vi "Manual_Cool_Heat.vi"(8 "error in":errorcluster, 11 "input cluster":T3={"Core"={"Current VI Reference"=refnum, "Close Panel on Exit?"=FALSE, "Exit"=FALSE, "Initialized?"=FALSE}, "Connections"={"cDAQ"={"Task"="", "Connected"=TRUE, "Active"=TRUE, "ID"=""}, "Camera"={"Session"="16511205", "Connected"=TRUE, "Active"=FALSE, "Placeholder"=refnum}, "PSU"={"Port"="", "Connected"=FALSE, "Active"=FALSE}, "Arduino"={"Port"="", "Connected"=FALSE, "Active"=FALSE}}, "Data Acquisition"={"Setup"={"Label"="Sample", "Operator"="N/A", "Notes"="", "TempGrad"=-1.0, "TargetTemp"=-30.0, "Sample Volume"=1.0}, "Camera"={"Image"=refnum, "Save Image"=refnum, "Image Frequency"=20, "Rectangle"={"Left"=163, "Top"=40, "Right"=1653, "Bottom"=1024, "Rotation"=0.0}, "Calibration"={"Top Left"={"X"=0.0, "Y"=0.0}, "Top Right"={"X"=0.0, "Y"=0.0}, "Bottom Left"={"X"=0.0, "Y"=0.0}, "Bottom Right"={"X"=0.0, "Y"=0.0}, "Fixpoint"={"X"=0.0, "Y"=0.0}, "Scan Area"=0.0, "Fixpoint Area"=0.0, "Well Pixels"=[], "Valid"=FALSE}, "FocusPos"=0, "Display Mapping"=10}, "Thermistor"={"Sample Size"=3, "Calibration"={"B0.100"=[3746.6, 3750.1, 3743.8, 3749.4, 3745.3, 3741.2, 3742.3, 3742.5], "R25"=[2.2535, 2.2652, 2.2631, 2.2631, 2.2631, 2.2501, 2.2549, 2.2676], "c"=[[-1.735921, 1.0956271, -0.2334593, 0.0229947, -0.0009224], [-2.1276337, 1.4006174, -0.3194056, 0.0337046, -0.0014085], [-2.1731341, 1.4499599, -0.3370628, 0.036201, -0.0015282], [-2.0647232, 1.3741488, -0.3194613, 0.0344214, -0.0014593], [-2.356994, 1.6319471, -0.3929067, 0.0428522, -0.0017977], [-2.0427871, 1.4165762, -0.345474, 0.0385267, -0.0016538], [-2.1725266, 1.4989325, -0.3661616, 0.0412033, -0.0017892], [-2.2048521, 1.4601067, -0.3370514, 0.0360935, -0.0015259]], "State"=[FALSE, TRUE, TRUE, TRUE, FALSE, FALSE, FALSE, FALSE], "V_S"=12.004, "R_S"=10.0}, "Timing Mode"=14713}, "Partition"={"Data"=[], "Cell Label"="", "Cell Color"=0, "Height"=10, "Width"=16, "Grid"=[]}, "Queue"={"Size"=10, "Queue"=refnum}, "Sample Rate"=120, "Active"=FALSE, "Ready"=TRUE, "Graph Mode"=0, "Gradient Buffer"=2}, "Control"={"Sample Rate"=1, "PID gains"={"proportional gain (Kc)"=7.56364319842873, "integral time (Ti, min)"=0.13615714612774, "derivative time (Td, min)"=0.0301129593449614}}, "Manual Temp Control"={"TargetTemp"=1.0, "Mode"=0, "Active"=FALSE}} {"Manual Temp Control"."Mode" items=["Cool", "Heat"]; "Manual Temp Control"."TargetTemp" min=-40.0 max=40.0 step=0.5 format="%#_g °C"; "Control"."PID gains"."derivative time (Td, min)" format="%.3f"; "Control"."PID gains"."integral time (Ti, min)" format="%.3f"; "Control"."PID gains"."proportional gain (Kc)" format="%.3f"; "Control"."Sample Rate" min=1 max=20 step=1 format="%.0f Samples/sec"; "Data Acquisition"."Gradient Buffer" min=2 max=30 step=1; "Data Acquisition"."Graph Mode" items=["Thermistor Temperature", "Camera Temperature"]; "Data Acquisition"."Thermistor"."Timing Mode" items=["Automatic"=16097, "High Resolution"=10195, "High Speed"=14712, "Best 50 Hz Rejection"=14713, "Best 60 Hz Rejection"=14714, "Custom"=10137]; "Data Acquisition"."Thermistor"."Calibration"."R_S" min=0.1 max=1000.0 format="%#_g kOhm"; "Data Acquisition"."Thermistor"."Calibration"."V_S" min=5.0 max=48.0 format="%#_g V"; "Data Acquisition"."Thermistor"."Calibration"."R25" min=0.1 max=1000.0 format="%#_g kOhm"; "Data Acquisition"."Thermistor"."Calibration"."B0.100" min=100.0 max=10000.0 format="%#_g K"; "Data Acquisition"."Thermistor"."Sample Size" min=1 max=200; "Data Acquisition"."Sample Rate" min=20 max=240 format="%.0f samples/min"; "Data Acquisition"."Queue"."Size" min=1 max=200; "Data Acquisition"."Camera"."Display Mapping" items=["Default"=10, "Most Significant Bits"=11, "Full Dynamic"=12, "Downshift"=13, "Given Range"=14, "90% Dynamic"=15, "Given Percent Range"=16]; "Data Acquisition"."Camera"."Calibration"."Fixpoint"."Y" format="%.2f"; "Data Acquisition"."Camera"."Calibration"."Fixpoint"."X" format="%.2f"; "Data Acquisition"."Camera"."Calibration"."Top Left"."Y" format="%.2f"; "Data Acquisition"."Camera"."Calibration"."Top Left"."X" format="%.2f"; "Data Acquisition"."Camera"."Calibration"."Top Right"."Y" format="%.2f"; "Data Acquisition"."Camera"."Calibration"."Top Right"."X" format="%.2f"; "Data Acquisition"."Camera"."Calibration"."Bottom Left"."Y" format="%.2f"; "Data Acquisition"."Camera"."Calibration"."Bottom Left"."X" format="%.2f"; "Data Acquisition"."Camera"."Calibration"."Bottom Right"."Y" format="%.2f"; "Data Acquisition"."Camera"."Calibration"."Bottom Right"."X" format="%.2f"; "Data Acquisition"."Camera"."Rectangle"."Rotation" min=-90.0 max=90.0 step=1.0 format="%.2f"; "Data Acquisition"."Camera"."Rectangle"."Left" scale=0.0..1024.0; "Data Acquisition"."Camera"."Rectangle"."Right" scale=0.0..1024.0; "Data Acquisition"."Camera"."Image Frequency" min=1 max=60 step=1; "Data Acquisition"."Setup"."Sample Volume" min=0.0 max=500.0 format="%#_g µL"; "Data Acquisition"."Setup"."TargetTemp" min=-40.0 max=40.0 step=0.5 format="%#_g °C"; "Data Acquisition"."Setup"."TempGrad" min=-100.0 max=100.0 step=0.1 format="%#_g °C/min"}) -> (0 "error out":errorcluster, 2 "State out":string, 3 "input cluster out":T3={"Core"={"Current VI Reference"=refnum, "Close Panel on Exit?"=FALSE, "Exit"=FALSE, "Initialized?"=FALSE}, "Connections"={"cDAQ"={"Task"="", "Connected"=TRUE, "Active"=TRUE, "ID"=""}, "Camera"={"Session"="16511205", "Connected"=TRUE, "Active"=FALSE, "Placeholder"=refnum}, "PSU"={"Port"="", "Connected"=FALSE, "Active"=FALSE}, "Arduino"={"Port"="", "Connected"=FALSE, "Active"=FALSE}}, "Data Acquisition"={"Setup"={"Label"="Sample", "Operator"="N/A", "Notes"="", "TempGrad"=-1.0, "TargetTemp"=-30.0, "Sample Volume"=1.0}, "Camera"={"Image"=refnum, "Save Image"=refnum, "Image Frequency"=20, "Rectangle"={"Left"=163, "Top"=40, "Right"=1653, "Bottom"=1024, "Rotation"=0.0}, "Calibration"={"Top Left"={"X"=0.0, "Y"=0.0}, "Top Right"={"X"=0.0, "Y"=0.0}, "Bottom Left"={"X"=0.0, "Y"=0.0}, "Bottom Right"={"X"=0.0, "Y"=0.0}, "Fixpoint"={"X"=0.0, "Y"=0.0}, "Scan Area"=0.0, "Fixpoint Area"=0.0, "Well Pixels"=[], "Valid"=FALSE}, "FocusPos"=0, "Display Mapping"=10}, "Thermistor"={"Sample Size"=3, "Calibration"={"B0.100"=[3746.6, 3750.1, 3743.8, 3749.4, 3745.3, 3741.2, 3742.3, 3742.5], "R25"=[2.2535, 2.2652, 2.2631, 2.2631, 2.2631, 2.2501, 2.2549, 2.2676], "c"=[[-1.735921, 1.0956271, -0.2334593, 0.0229947, -0.0009224], [-2.1276337, 1.4006174, -0.3194056, 0.0337046, -0.0014085], [-2.1731341, 1.4499599, -0.3370628, 0.036201, -0.0015282], [-2.0647232, 1.3741488, -0.3194613, 0.0344214, -0.0014593], [-2.356994, 1.6319471, -0.3929067, 0.0428522, -0.0017977], [-2.0427871, 1.4165762, -0.345474, 0.0385267, -0.0016538], [-2.1725266, 1.4989325, -0.3661616, 0.0412033, -0.0017892], [-2.2048521, 1.4601067, -0.3370514, 0.0360935, -0.0015259]], "State"=[FALSE, TRUE, TRUE, TRUE, FALSE, FALSE, FALSE, FALSE], "V_S"=12.004, "R_S"=10.0}, "Timing Mode"=14713}, "Partition"={"Data"=[], "Cell Label"="", "Cell Color"=0, "Height"=10, "Width"=16, "Grid"=[]}, "Queue"={"Size"=10, "Queue"=refnum}, "Sample Rate"=120, "Active"=FALSE, "Ready"=TRUE, "Graph Mode"=0, "Gradient Buffer"=2}, "Control"={"Sample Rate"=1, "PID gains"={"proportional gain (Kc)"=7.56364319842873, "integral time (Ti, min)"=0.13615714612774, "derivative time (Td, min)"=0.0301129593449614}}, "Manual Temp Control"={"TargetTemp"=1.0, "Mode"=0, "Active"=FALSE}} {"Manual Temp Control"."Mode" items=["Cool", "Heat"]; "Manual Temp Control"."TargetTemp" min=-40.0 max=40.0 step=0.5 format="%#_g °C"; "Control"."PID gains"."derivative time (Td, min)" format="%.3f"; "Control"."PID gains"."integral time (Ti, min)" format="%.3f"; "Control"."PID gains"."proportional gain (Kc)" format="%.3f"; "Control"."Sample Rate" min=1 max=20 step=1 format="%.0f Samples/sec"; "Data Acquisition"."Gradient Buffer" min=2 max=30 step=1; "Data Acquisition"."Graph Mode" items=["Thermistor Temperature", "Camera Temperature"]; "Data Acquisition"."Thermistor"."Timing Mode" items=["Automatic"=16097, "High Resolution"=10195, "High Speed"=14712, "Best 50 Hz Rejection"=14713, "Best 60 Hz Rejection"=14714, "Custom"=10137]; "Data Acquisition"."Thermistor"."Calibration"."R_S" min=0.1 max=1000.0 format="%#_g kOhm"; "Data Acquisition"."Thermistor"."Calibration"."V_S" min=5.0 max=48.0 format="%#_g V"; "Data Acquisition"."Thermistor"."Calibration"."R25" min=0.1 max=1000.0 format="%#_g kOhm"; "Data Acquisition"."Thermistor"."Calibration"."B0.100" min=100.0 max=10000.0 format="%#_g K"; "Data Acquisition"."Thermistor"."Sample Size" min=1 max=200; "Data Acquisition"."Sample Rate" min=20 max=240 format="%.0f samples/min"; "Data Acquisition"."Queue"."Size" min=1 max=200; "Data Acquisition"."Camera"."Display Mapping" items=["Default"=10, "Most Significant Bits"=11, "Full Dynamic"=12, "Downshift"=13, "Given Range"=14, "90% Dynamic"=15, "Given Percent Range"=16]; "Data Acquisition"."Camera"."Calibration"."Fixpoint"."Y" format="%.2f"; "Data Acquisition"."Camera"."Calibration"."Fixpoint"."X" format="%.2f"; "Data Acquisition"."Camera"."Calibration"."Top Left"."Y" format="%.2f"; "Data Acquisition"."Camera"."Calibration"."Top Left"."X" format="%.2f"; "Data Acquisition"."Camera"."Calibration"."Top Right"."Y" format="%.2f"; "Data Acquisition"."Camera"."Calibration"."Top Right"."X" format="%.2f"; "Data Acquisition"."Camera"."Calibration"."Bottom Left"."Y" format="%.2f"; "Data Acquisition"."Camera"."Calibration"."Bottom Left"."X" format="%.2f"; "Data Acquisition"."Camera"."Calibration"."Bottom Right"."Y" format="%.2f"; "Data Acquisition"."Camera"."Calibration"."Bottom Right"."X" format="%.2f"; "Data Acquisition"."Camera"."Rectangle"."Rotation" min=-90.0 max=90.0 step=1.0 format="%.2f"; "Data Acquisition"."Camera"."Rectangle"."Left" scale=0.0..1024.0; "Data Acquisition"."Camera"."Rectangle"."Right" scale=0.0..1024.0; "Data Acquisition"."Camera"."Image Frequency" min=1 max=60 step=1; "Data Acquisition"."Setup"."Sample Volume" min=0.0 max=500.0 format="%#_g µL"; "Data Acquisition"."Setup"."TargetTemp" min=-40.0 max=40.0 step=0.5 format="%#_g °C"; "Data Acquisition"."Setup"."TempGrad" min=-100.0 max=100.0 step=0.1 format="%#_g °C/min"})   [LabVIEW 2022 SP3]
uses:
  DataCluster.ctl
  <vilib>/userdefined/High Color/IMAQdx.ctl
  <vilib>/vision/Image Controls.llb/IMAQ Image.ctl
  <vilib>/addons/control/pid/autopid.llb/PID autotuning parameters (FO).ctl
  <vilib>/Platform/TimedLoop/XDataNode/timing_clust.ctl
  <vilib>/Platform/TimedLoop/XDataNode/nitl_modes.ctl
  <vilib>/Platform/TimedLoop/XDataNode/wakeup.ctl
  3b4f4478-d76b-4d41-92af-3e1abf8851fc.vi
  <extravilib>/ChannelInstances/Tag-bool/Write With Abort.vi
  <extravilib>/ChannelInstances/Tag-bool/Read With Abort.vi
  <extravilib>/ChannelInstances/Tag-bool/Instantiate.vi
  <extravilib>/ChannelInstances/Tag-bool/EndpointRead.vi
  <extravilib>/ChannelInstances/Tag-bool/Endpoint.vi
  <vilib>/platform/TimedLoop/XDataNode/XDataNode.xnode
  <vilib>/Platform/TimedLoop/XDataNode/XDNodeRunTimeDep.lvlib
  <extravilib>/ChannelInstances/Tag-bool.lvlib
  <vilib>/addons/control/pid/NI_PID_autopid.lvlib
panel:
  in  "Target Temp":dbl=-30.0 min=-30.0 max=50.0 step=0.5 format="%#_g °C"
  in  "Start":bool
  out "Output%":dbl(slide) caption="Cooling" scale=0.0..100.0 scale format="%#_g %"
  in  "Auto PID":enum32{"Results", "Setup"}(tab)
  out "plant parameters":T1={"process gain"=1.0, "time constant (s)"=0.01, "delay time (s)"=0.0}
  in  "Accept Values":bool
  in  "Auto_param":T2={"type of controller"=2, "time constant factor"=1.0, "step amplitude"=15.0} {"step amplitude" format="%.2f"; "type of controller" items=["P", "PI", "PID"]}
  in  "beta":dbl=1.0 format="%.2f"
  in  "alpha":dbl=0.1 format="%.2f"
  in  "Auto PID":bool
  in  "Target Gradient":dbl=-1.0 min=-100.0 max=100.0 step=0.1 format="%#_g °C/min"
  in  "Derivative time":dbl=0.0301129593449614 min=0.0 format="%.3f min"
  in  "Integral time":dbl=0.13615714612774 min=0.0 format="%.3f min"
  in  "Proportional gain":dbl=7.56364319842873 min=0.0 format="%.3f"
  out "Gradients":waveform(dbl)[](graph)=[{"t0"=timestamp(0 s since 1904-01-01), "dt"=0.5, "Y"=[7.433224549329398, 0.895625095359529, 0.9552816832532773, 0.9304725526031321, 0.9043782200494332, 0.9306810462591653, 0.8938101718101077, 0.925790375665021, 0.9288831091681904, 0.9008028671153312, 0.9156395957693197, 0.9226399096000337, 0.8971103852841011, 0.9108706371930864, 0.9015980851396677, 0.9063524311916105, 0.8952556646095977, 0.917940923503271, 0.8923980038918522, 0.8956796305886883, 0.8903847671434284, 0.9062834028185462, 0.8780323964554282, 0.9015016131968667, 0.9254937279973241, 0.8669157938798877, 0.8811376124795678, 0.8809039296201449, 0.8673280290474628, 0.8900629488959377, 0.8803663660038574, 0.8752191981067758, 0.8814481119261552, 0.8171494045248751, 0.875717028408618, 0.8513436228943982, 0.852814524743839, 0.8575626914160073, 0.8751490584860311, 0.850681612810047, 0.8235316783120428, 0.8337861461206697, 0.8623430055829617, 0.8450758215557541, 0.8373026615072277, 0.8144489454929282, 0.8152893746080092, 0.8315843982206106, 0.8276838319805702, 0.8150641369387401, 0.8002372598659058, 0.8087715632678205, 0.7895667029526843, 0.8137766484500419, 0.8207441169410812, 0.7380692415395407, 0.7987438003888592, 0.7747114976546943, 0.7873097270606588, 0.7741697534382058, 0.7392447124350643, 0.7674326823990801, 0.758637239692122, 0.7678967997914032, 0.7265900533383629, 0.7564921061289931, 0.729315990067137, 0.7334050593326014, 0.7312180058105167, 0.6981534879929185, 0.7390729137931951, 0.7027665547718651, 0.6968681528036582]}, {"t0"=timestamp(0 s since 1904-01-01), "dt"=0.5, "Y"=[-1.0, -1.0, -1.0, -1.0, -1.0, -1.0, -1.0, -1.0, -1.0, -1.0, -1.0, -1.0, -1.0, -1.0, -1.0, -1.0, -1.0, -1.0, -1.0, -1.0, -1.0, -1.0, -1.0, -1.0, -1.0, -1.0, -1.0, -1.0, -1.0, -1.0, -1.0, -1.0, -1.0, -1.0, -1.0, -1.0, -1.0, -1.0, -1.0, -1.0, -1.0, -1.0, -1.0, -1.0, -1.0, -1.0, -1.0, -1.0, -1.0, -1.0, -1.0, -1.0, -1.0, -1.0, -1.0, -1.0, -1.0, -1.0, -1.0, -1.0, -1.0, -1.0, -1.0, -1.0, -1.0, -1.0, -1.0, -1.0, -1.0, -1.0, -1.0, -1.0, -1.0]}]
  out "Temps":waveform(dbl)[](graph)=[{"t0"=timestamp(0 s since 1904-01-01), "dt"=0.5, "Y"=[-0.5459297948238789, -0.5384662523625495, -0.5305055716687722, -0.5227516337304128, -0.5152151485633342, -0.5074594731778411, -0.5000110550794236, -0.49229613528221505, -0.48455544270581347, -0.47704875214651904, -0.4694184221817747, -0.4617297562684411, -0.4542538363910736, -0.44666324774779786, -0.43914993037163397, -0.4315969934450372, -0.42413652957329057, -0.41648702187743, -0.4090503718449979, -0.40158637492342547, -0.3941665018638969, -0.38661414017374235, -0.3792972035366138, -0.37178469009330656, -0.3640722423599955, -0.3568479440776631, -0.3495051306403334, -0.3421642645601655, -0.33493653098477, -0.3275193397439705, -0.32018295336060504, -0.3128894600430486, -0.3055440591103306, -0.29873448073929, -0.29143683883588484, -0.2843423086450982, -0.2772355209388995, -0.27008916517709947, -0.26279625635638254, -0.2557072429162988, -0.24884447893036513, -0.2418962610460262, -0.23471006933283486, -0.22766777081987025, -0.22069024864064335, -0.21390317409486895, -0.20710909597313554, -0.20017922598796378, -0.19328186072145903, -0.18648965958030286, -0.17982101574808698, -0.17308125272085514, -0.16650153019624944, -0.15972005812583243, -0.15288052381799008, -0.14672994680516058, -0.14007374846858675, -0.1336178193214643, -0.12705690492929214, -0.12060549031730709, -0.11444511771368156, -0.10804984536035589, -0.10172786836292154, -0.09532872836465985, -0.08927381125350682, -0.08296971036909855, -0.07689207711853907, -0.07078036829076739, -0.06468688490901309, -0.058868939175738766, -0.05270999822746214, -0.04685361027102993, -0.04104637566433278]}, {"t0"=timestamp(0 s since 1904-01-01), "dt"=0.5, "Y"=[-30.0, -30.0, -30.0, -30.0, -30.0, -30.0, -30.0, -30.0, -30.0, -30.0, -30.0, -30.0, -30.0, -30.0, -30.0, -30.0, -30.0, -30.0, -30.0, -30.0, -30.0, -30.0, -30.0, -30.0, -30.0, -30.0, -30.0, -30.0, -30.0, -30.0, -30.0, -30.0, -30.0, -30.0, -30.0, -30.0, -30.0, -30.0, -30.0, -30.0, -30.0, -30.0, -30.0, -30.0, -30.0, -30.0, -30.0, -30.0, -30.0, -30.0, -30.0, -30.0, -30.0, -30.0, -30.0, -30.0, -30.0, -30.0, -30.0, -30.0, -30.0, -30.0, -30.0, -30.0, -30.0, -30.0, -30.0, -30.0, -30.0, -30.0, -30.0, -30.0, -30.0]}]
  out "Status":string="System ready"
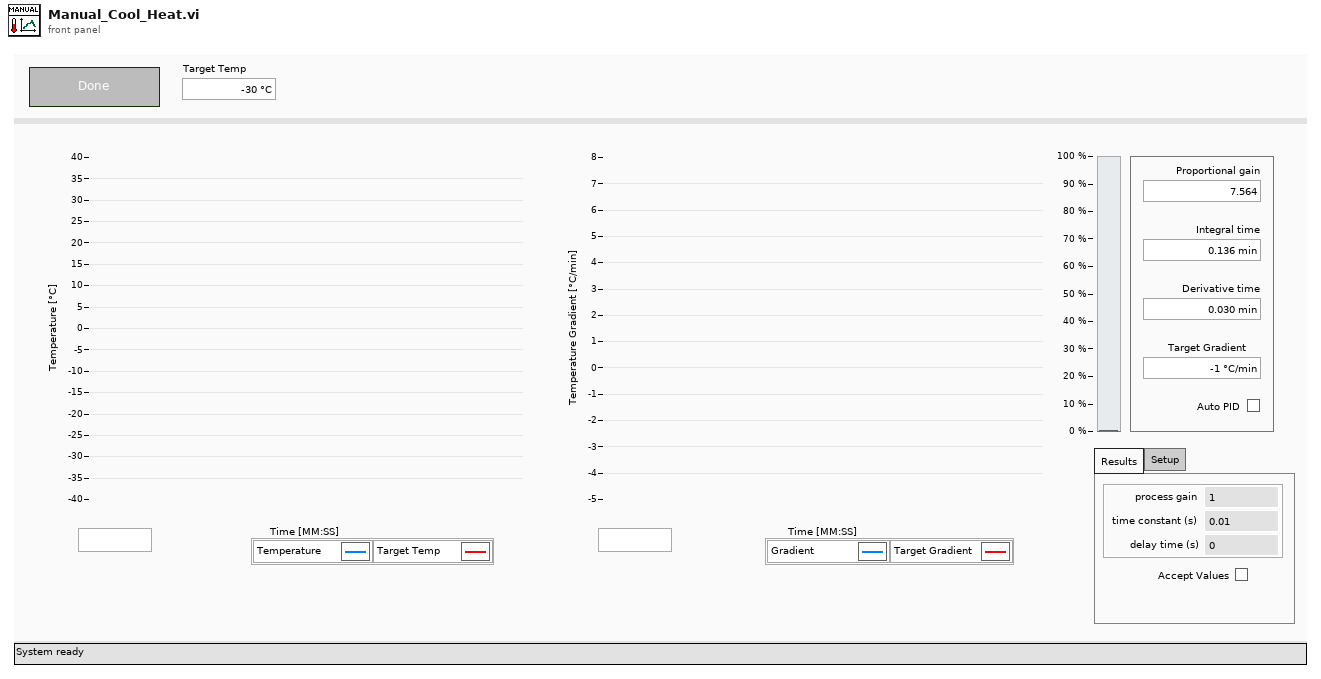
[diagram p1: front panel]
types:
  T1 = cluster{"process gain":dbl, "time constant (s)":dbl, "delay time (s)":dbl}
  T2 = typedef "NI_PID_autopid.lvlib/PID autotuning parameters (FO).ctl" = cluster{"type of controller":u16, "time constant factor":dbl, "step amplitude":dbl}
  T3 = typedef "DataCluster.ctl" = cluster{"Core":cluster{"Current VI Reference":refnum<vi>, "Close Panel on Exit?":bool, "Exit":bool, "Initialized?":bool}, "Connections":cluster{"cDAQ":cluster{"Task":refnum<k21>, "Connected":bool, "Active":bool, "ID":string}, "Camera":cluster{"Session":T4, "Connected":bool, "Active":bool, "Placeholder":T5}, "PSU":cluster{"Port":refnum<visa-resource-name>, "Connected":bool, "Active":bool}, "Arduino":cluster{"Port":refnum<visa-resource-name>, "Connected":bool, "Active":bool}}, "Data Acquisition":cluster{"Setup":cluster{"Label":string, "Operator":string, "Notes":string, "TempGrad":dbl, "TargetTemp":dbl, "Sample Volume":dbl}, "Camera":cluster{"Image":T5, "Save Image":T5, "Image Frequency":i32, "Rectangle":T6, "Calibration":cluster{"Top Left":T7, "Top Right":T7, "Bottom Left":T7, "Bottom Right":T7, "Fixpoint":T7, "Scan Area":dbl, "Fixpoint Area":dbl, "Well Pixels":cluster{"X":i32, "Y":i32}[][], "Valid":bool}, "FocusPos":u32, "Display Mapping":u32}, "Thermistor":cluster{"Sample Size":i32, "Calibration":cluster{"B0.100":dbl[], "R25":dbl[], "c":dbl[][], "State":bool[], "V_S":dbl, "R_S":dbl}, "Timing Mode":i32}, "Partition":cluster{"Data":string[][], "Cell Label":string, "Cell Color":u32, "Height":i32, "Width":i32, "Grid":string[][]}, "Queue":cluster{"Size":i32, "Queue":refnum<queue>}, "Sample Rate":i32, "Active":bool, "Ready":bool, "Graph Mode":u16, "Gradient Buffer":i32}, "Control":cluster{"Sample Rate":i32, "PID gains":cluster{"proportional gain (Kc)":dbl, "integral time (Ti, min)":dbl, "derivative time (Td, min)":dbl}}, "Manual Temp Control":cluster{"TargetTemp":dbl, "Mode":u16, "Active":bool}}
  T4 = typedef "IMAQdx.ctl" = refnum<k21>
  T5 = typedef "IMAQ Image.ctl" = refnum<image>
  T6 = typedef "IMAQ Rectangle" = cluster{"Left":i32, "Top":i32, "Right":i32, "Bottom":i32, "Rotation":dbl}
  T7 = typedef "IMAQ Point" = cluster{"X":sgl, "Y":sgl}
  T8 = typedef "Tag-bool.lvlib/))Channel.ctl" = refnum<queue>
  T9 = enum8{"Enabled", "Disabled", "Disabled and Grayed Out"}
  T10 = typedef "XDNodeRunTimeDep.lvlib/timing_clust.ctl" = cluster{"Expected End [f-1]":u64, "Actual End [f-1]":u64, "Finished Late? [f-1]":bool, "Expected End [i-1]":u64, "Actual End [i-1]":u64, "Finished Late? [i-1]":bool, "Expected Start [i]":u64, "Actual Start [i]":u64, "Expected Start [f]":u64, "Actual Start [f]":u64, "Source Name":string, "Structure Name":string, "Period":i64, "Deadline":i64, "Offset":i64, "Start":i64, "Priority":i32, "Timeout":i32, "Mode":T11, "Wakeup Reason":T12, "Error":errorcluster, "Source Type":string, "Secondary Source Type":string, "Global End Time":u64, "Global Start Time":u64, "Frame Duration":u64, "Iteration Duration":u64, "Assigned CPU":i32, "I/O Scan Engine Mode":u32}
  T11 = typedef "XDNodeRunTimeDep.lvlib/nitl_modes.ctl" = enum32{"No Change", "Process missed periods, maintain original phase", "Discard missed periods, maintain original phase", "Process missed periods, ignore original phase", "Discard missed periods, ignore original phase"}
  T12 = typedef "XDNodeRunTimeDep.lvlib/wakeup.ctl" = enum32{"Normal", "Aborted", "Asynchronous wakeup", "Timing source error", "Timed loop error", "Timeout"}
  T13 = cluster{"proportional gain (Kc)":dbl, "integral time (Ti, min)":dbl, "derivative time (Td, min)":dbl}
  T14 = cluster{"Proportional gain":dbl, "Integral time ":dbl, "Derivative time":dbl}
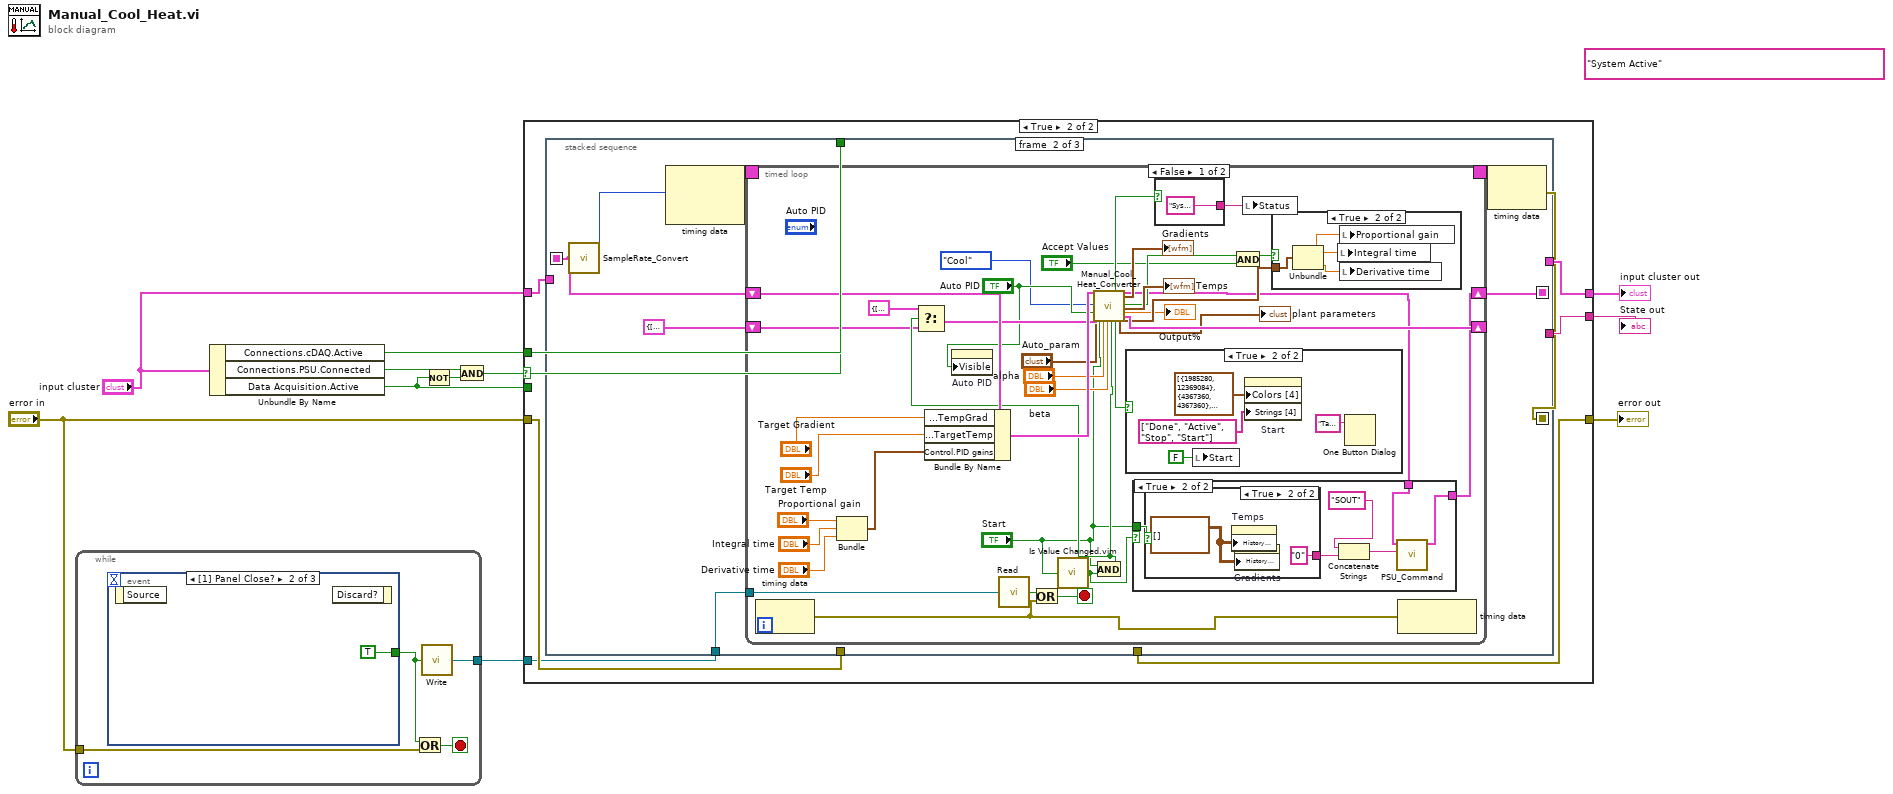
[diagram p0: block diagram]
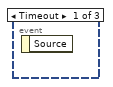
[diagram p2: hidden frame]
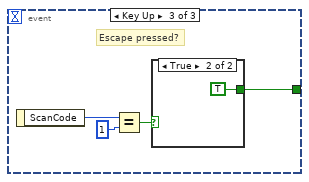
[diagram p3: hidden frame]
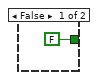
[diagram p4: hidden frame]
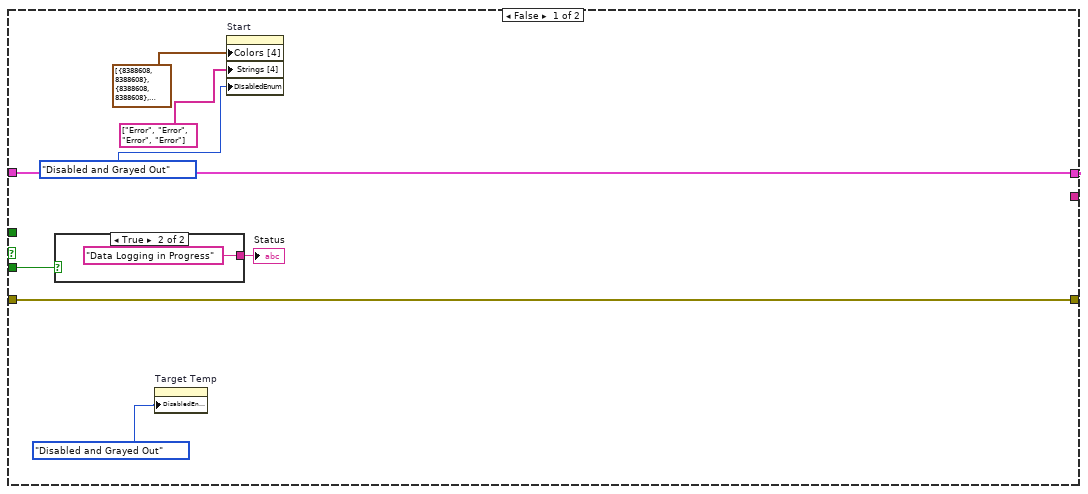
[diagram p5: hidden frame]
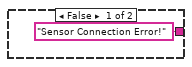
[diagram p6: hidden frame]
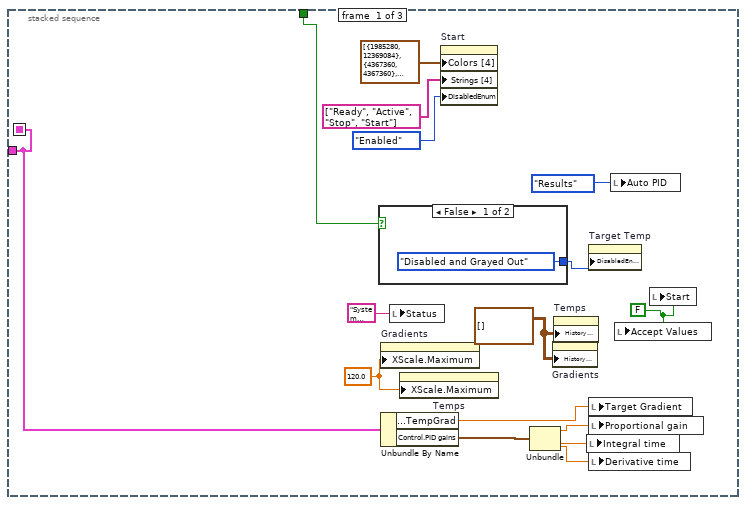
[diagram p7: hidden frame]
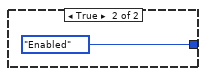
[diagram p8: hidden frame]
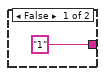
[diagram p11: hidden frame]
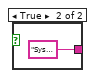
[diagram p13: hidden frame]
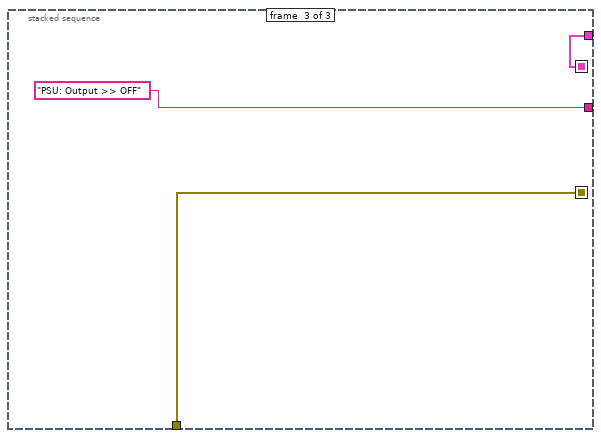
[diagram p14: hidden frame]
diagram:
  (unwired) "System Active" ("Status")
  n1 = while {
    tunnel: "error in" -> [w13]
    tunnel: [w12] -> w9
    stop <- w14 stop-if-true
    n2 = event shown="[1] Panel Close?" {
      selector: _ -> [_ _ _]
      dyn-events: _ -> [_ _ _]
      timeout: _ -> [_ _ _]
      tunnel: [_ TRUE w20] -> w15
      event Timeout {
        n3 = event-data() -> ()  [unwired: 1 in, 1 out]
      }
      event Panel Close? {
        n4 = event-data() -> ()  [unwired: 1 in, 1 out]
        n5 = event-data() -> ()  [unwired: 2 in, 1 out]
      }
      event Key Up {
        # "Escape pressed?"
        n6 = event-data() -> ("ScanCode"=w19:i16)  [unwired: 1 in]
        n7 = Equal?(x=w19, y=i16 1) -> (x = y?=w17:bool)
        n8 = case shown="True" w17 {
          tunnel: [FALSE TRUE] -> w20
          frame False {
          }
          frame True {
          }
        }
      }
    }
    n9 = Or(x=w15, y=w13) -> (x .or. y?=w14:bool)
    n10 = call <extravilib>:"Write.vi"("element"=w15) -> ("channel"=w12:T8)  [unwired: 1 out]
  }
  n11 = Unbundle By Name("input cluster") -> ("Connections.cDAQ.Active"=w7:bool, "Connections.PSU.Connected"=w6:bool, "Data Acquisition.Active"=w3:bool)
  n12 = Not(x=w3) -> (.not. x?=w4:bool)
  n13 = And(x=w6, y=w4) -> (x .and. y?=w5:bool)
  n14 = case shown="True" w5 {
    selector: w5 -> [_ w34]
    tunnel: "error in" -> [w30 w40]
    tunnel: [w30 w39] -> w11
    tunnel: w9 -> [_ w38]
    tunnel: "input cluster" -> [w24 w37]
    tunnel: w7 -> [_ w36]
    tunnel: w3 -> [w25 _]
    tunnel: [w24 w35] -> w2
    tunnel: [_ w33] -> w1
    frame False {
      n15 = case shown="True" w25 {
        tunnel: ["Sensor Connection Error!" ("String") "Data Logging in Progress" ("String")] -> w29
        frame False {
        }
        frame True {
        }
      }
      "Status" <- w29
      n16 = property on="Target Temp" class="DigNum (strict)"("DisabledEnum"=T9."Disabled and Grayed Out" ("Disabled")) -> ()  [unwired: 2 in, 2 out]
      n17 = property on="Start" class="Bool (strict)"("Colors [4]"=cluster{u32, u32}[] [{8388608, 8388608}, {8388608, 8388608}, {8388608, 8388608}, {8388608, 8388608}, {8388608, 8388608}, {16711681, 16711680}], "Strings [4]"=string[] ["Error", "Error", "Error", "Error"], "DisabledEnum"=T9."Disabled and Grayed Out" ("Disabled")) -> ()  [unwired: 2 in, 2 out]
    }
    frame True {
      n18 = stacked-sequence {
        seq-local: [w51 _ _] -> [_ w62 _]
        seq-local: [_ w63 _] -> [_ _ w136]
        seq-local: [_ w59 _] -> [_ _ w135]
        tunnel: w40 -> [_ _ _]
        tunnel: w37 -> [w51 _ _]
        tunnel: w36 -> [_ _ _]
        tunnel: w34 -> [w42 _ _]
        tunnel: w38 -> [_ w66 _]
        tunnel: [_ _ w136] -> w39
        tunnel: [_ _ w135] -> w35
        tunnel: [_ _ "PSU: Output >> OFF"] -> w33
        frame #0 {
          w43 = 120.0 ("X Scale.Range:Maximum")
          w41 = FALSE ("Accept Values")
          w52 = waveform(dbl)[][] [] ("History Data")
          n19 = case shown="False" w42 {
            tunnel: [T9."Disabled and Grayed Out" ("Disabled") T9."Enabled" ("Disabled")] -> w45
            frame False {
            }
            frame True {
            }
          }
          n20 = property on="Gradients" class="WFChart (strict)"("XScale.Maximum"=w43) -> ()  [unwired: 2 in, 2 out]
          n21 = Unbundle By Name(w51) -> ("Data Acquisition.Setup.TempGrad"=w46:dbl, "Control.PID gains"=w50:T13)
          n22 = local write "Status"("System Ready" ("Status")) -> ()
          n23 = property on="Temps" class="WFChart (strict)"("XScale.Maximum"=w43) -> ()  [unwired: 2 in, 2 out]
          n24 = property on="Start" class="Bool (strict)"("Colors [4]"=cluster{u32, u32}[] [{1985280, 12369084}, {4367360, 4367360}, {8388608, 16711681}, {1985280, 1985280}, {1985280, 4367360}, {8388608, 16711681}], "Strings [4]"=string[] ["Ready", "Active", "Stop", "Start"], "DisabledEnum"=T9."Enabled" ("Disabled")) -> ()  [unwired: 2 in, 2 out]
          n25 = Unbundle(w50) -> ("proportional gain (Kc)"=w49:dbl, "integral time (Ti, min)"=w48:dbl, "derivative time (Td, min)"=w47:dbl)
          n26 = property on="Gradients" class="WFChart (strict)"("History Data"=w52) -> ()  [unwired: 2 in, 2 out]
          n27 = property on="Temps" class="WFChart (strict)"("History Data"=w52) -> ()  [unwired: 2 in, 2 out]
          n28 = local write "Integral time"(w48) -> ()
          n29 = property on="Target Temp" class="DigNum (strict)"("DisabledEnum"=w45) -> ()  [unwired: 2 in, 2 out]
          n30 = local write "Target Gradient"(w46) -> ()
          n31 = local write "Proportional gain"(w49) -> ()
          n32 = local write "Derivative time"(w47) -> ()
          n33 = local write "Auto PID"(enum32{"Results", "Setup"}."Results" ("Auto PID")) -> ()
          n34 = local write "Accept Values"(w41) -> ()
          n35 = local write "Start"(w41) -> ()
        }
        frame #1 {
          n36 = call "SampleRate_Convert.vi"("DataCluster"=w62) -> ("Sample dt (ms)"=w60:i64)  [unwired: 1 out]
          n37 = node-c288(w60) -> (w65:T10)  [unwired: 1 in]
          n38 = timed-loop {
            tunnel: w66 -> [w102]
            timing: w65 -> [_]
            timing-out: [_] -> w64
            shift-right: [w97] -> _
            shift-left: cluster{dbl[], dbl[], dbl[], dbl[], dbl[][]} {[], [], [], [], []} ("Data Cluster in") -> [w84]
            shift-right: [w68] -> w59
            shift-left: w62 -> [w94]
            stop <- w103 stop-if-true
            n39 = node-c288() -> (w95:errorcluster)  [unwired: 1 in]
            n40 = Bundle("Proportional gain"="Proportional gain", "Integral time"="Integral time", "Derivative time"="Derivative time") -> (w88:T14)  [unwired: 1 in]
            n41 = Bundle By Name(cluster=w94, "Data Acquisition.Setup.TempGrad"="Target Gradient", "Data Acquisition.Setup.TargetTemp"="Target Temp", "Control.PID gains"=w88) -> (w93:T3)
            n42 = property on="Auto PID" class="TabCtl (strict)"("Visible"="Auto PID") -> ()  [unwired: 2 in, 2 out]
            n43 = call <extravilib>:"Read.vi"("channel"=w102) -> ("element"=w101:bool)  [unwired: 1 in, 1 out]
            n44 = Or(x=w101, y=w95) -> (x .or. y?=w103:bool)
            n45 = call "Is Value Changed.vim"("value"="Start") -> ("changed or first call?"=w71:bool)
            n46 = And(x="Start", y=w71) -> (x .and. y?=w85:bool)
            n47 = Select(t=cluster{dbl[], dbl[], dbl[], dbl[], dbl[][]} {[], [], [], [], []} ("Data Cluster in"), s=w85, f=w84) -> (s? t:f=w86:cluster{dbl[], dbl[], dbl[], dbl[], dbl[][]})
            n48 = call "Manual_Cool_Heat_Converter.vi"("input cluster"=w93, "Cool/Heat"=enum32{"Cool", "Heat"}."Cool", "Auto PID"="Auto PID", "autotuning parameters"="Auto_param", "Data Cluster in"=w86, "active?"="Start", "alpha"="alpha", "beta"="beta", "reinitialize? (F)"=w85) -> ("Active?"=w100:bool, "Temp Reached"=w98:bool, "plant parameters out"=→"plant parameters":T1, "input cluster out"=w69:T3, "Gradients"=→"Gradients":waveform(dbl)[], "tuning completed?"=w82:bool, "Temps"=→"Temps":waveform(dbl)[], "Output%"=→"Output%":dbl, "Data Cluster out"=w97:cluster{dbl[], dbl[], dbl[], dbl[], dbl[][]}, "PID gains out"=w81:T13)  [unwired: 9 in]
            n49 = case shown="True" w98 {
              frame False {
              }
              frame True {
                n50 = local write "Start"(FALSE ("Key Focus")) -> ()
                n51 = property on="Start" class="Bool (strict)"("Colors [4]"=cluster{u32, u32}[] [{1985280, 12369084}, {4367360, 4367360}, {8388608, 16711681}, {1985280, 1985280}, {1985280, 4367360}, {8388608, 16711681}], "Strings [4]"=string[] ["Done", "Active", "Stop", "Start"]) -> ()  [unwired: 2 in, 2 out]
                n52 = One Button Dialog(message="Target temperature reached.") -> ()  [unwired: 1 in, 1 out]
              }
            }
            n53 = case shown="True" w71 {
              tunnel: "Start" -> [_ w113]
              tunnel: w69 -> [w108 w111]
              tunnel: [w108 w110] -> w68
              frame False {
              }
              frame True {
                n54 = case shown="True" w113 {
                  tunnel: ["1" ("string") "0" ("string")] -> w112
                  frame False {
                  }
                  frame True {
                    w116 = waveform(dbl)[][] [] ("History Data")
                    n55 = property on="Temps" class="WFChart (strict)"("History Data"=w116) -> ()  [unwired: 2 in, 2 out]
                    n56 = property on="Gradients" class="WFChart (strict)"("History Data"=w116) -> ()  [unwired: 2 in, 2 out]
                  }
                }
                n57 = Concatenate Strings("SOUT" ("string"), w112) -> (w109:string)
                n58 = call "PSU_Command.vi"("command"=w109, "DataCluster"=w111) -> ("DataCluster out"=w110:T3)  [unwired: 7 in, 2 out]
              }
            }
            n59 = case shown="False" w100 {
              tunnel: ["System ready" ("Status") "System Active" ("Status")] -> w99
              frame False {
              }
              frame True {
              }
            }
            n60 = And(x=w82, y="Accept Values") -> (x .and. y?=w80:bool)
            n61 = local write "Status"(w99) -> ()
            n62 = case shown="True" w80 {
              tunnel: w81 -> [_ w107]
              frame False {
              }
              frame True {
                n63 = Unbundle(w107) -> ("proportional gain (Kc)"=w106:dbl, "integral time (Ti, min)"=w105:dbl, "derivative time (Td, min)"=w104:dbl)
                n64 = local write "Integral time"(w105) -> ()
                n65 = local write "Proportional gain"(w106) -> ()
                n66 = local write "Derivative time"(w104) -> ()
              }
            }
            n67 = node-c288(w95) -> ()  [unwired: 1 out]
          }
          n68 = node-c288(w64) -> (w63:errorcluster)
        }
        frame #2 {
        }
      }
    }
  }
  "error out" <- w11
  "input cluster out" <- w2
  "State out" <- w1
